vi "XIPIN_Peak_Cancellation_Crest_Factor_Reduction_3_0.vi"   [LabVIEW 2017]
doc: "The Peak Cancellation Crest Factor Reduction LogiCORE(TM) provides a flexible and highly efficient solution to reduce the peak to average power ratio (PAR) of complex multi-carrier waveforms.\n------------------------------------\n<b>Need License</b> : Yes\n<b>Interface</b> : AXI4-Stream AXI4-Lite"
uses:
  <vilib>/rvi/XilinxIP/XIPIN_XNode/niFpgaXIPIN.xnode
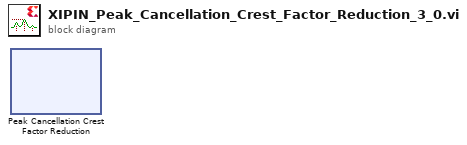
[diagram p0: block diagram]
diagram:
  n1 = xnode ("Peak Cancellation Crest Factor Reduction")() -> ()
